vi "Catalytic Methanation #1.vi"() -> ()   [LabVIEW 2017]
uses:
  Halt S&THx.vi
  <vilib>/addons/control/pid/pid.llb/PID Advanced (DBL).vi
  <vilib>/addons/control/pid/NI_PID_pid.lvlib
panel:
  out "Last Time Write":dbl
  in  "Replace File":bool
  in  "Recording Increment (sec)":dbl=0.3 min=0.1 max=100.0 step=0.1 format="%#_13g"
  in  "Enable 5":bool
  in  "stop":bool
  out "error constant":errorcluster
  out "Inlet Valve":bool=TRUE
  out "Heater On?":bool
  in  "Td (Pressure)":dbl
  in  "Ti (Pressure)":dbl=0.01
  in  "Kc (Pressure)":dbl=-5.0
  in  "Td (Heater)":dbl caption="(min)"
  in  "Ti (Heater)":dbl=5.0 caption="(min)"
  in  "Kc (Heater)":dbl=1.0
  in  "Select GC Analysis Stream":enum32{"Reactor Feed", "Reactor Exhaust"}(radio)=enum."Reactor Exhaust"
  out "He Flowrate (SCCM)":dbl format="%.1f"
  out "H2 Flowrate (SCCM)":dbl format="%.2f"
  out "CO2 Flowrate (SCCM)":dbl format="%.2f"
  in  "He Setpoint (SCCM)":dbl min=0.0 max=200.0 format="%.1f"
  in  "H2 Setpoint (SCCM)":dbl min=0.0 max=50.0 format="%.2f"
  in  "Heater Switch":bool
  in  "CO2 Setpoint (SCCM)":dbl min=0.0 max=10.0 format="%.2f"
  in  "Temperature Setpoint (C)":dbl=20.0 min=0.0 max=325.0 format="%.1f"
  out "Reactor Temperature (C)":dbl format="%.2f"
  out "Heater Output (%)":dbl(slide) scale=0.0..100.0
  in  "Manual  Override (Temperature)":bool=TRUE
  in  "Set Manual  Heater Output (Temperature)":dbl(slide) scale=0.0..100.0
  in  "Reactor Pressure  Setpoint (psia)":dbl=18.4 min=0.0 max=30.0 format="%.1f"
  out "Reactor Pressure (psia)":dbl format="%.1f"
  out "Pressure Control Valve (%)":dbl(slide) scale=0.0..100.0
  in  "Manual Override (Pressure)":bool=TRUE
  in  "Set Manual Valve Position (Pressure)":dbl(slide)=50.0 scale=0.0..100.0
  # "Heater Power"
  # "Total Flow > 190 SCCM\nH2/CO2 > 3.85\nGC Sample Path: Reactor Exhaust"
  # "Heater Control"
  # "Gas Flow Rates (SCCM)"
  # "Setpoint"
  # "Actual"
  # "Hydrogen"
  # "Carbon Dioxide"
  # "Helium"
  # "Data Collection"
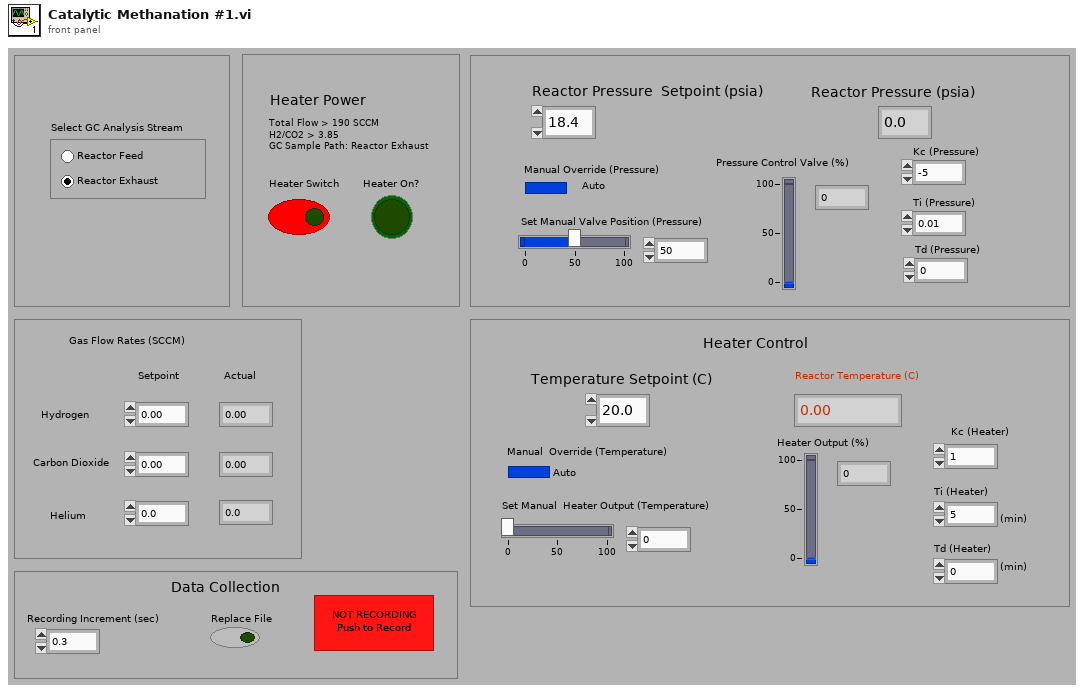
[diagram p1: front panel]
types:
  T1 = enum16{"open", "replace", "create", "open or create", "replace or create", "replace or create with confirmation"}
  T2 = cluster{"Kc (Heater)":dbl, "Ti (Heater)":dbl, "Td (Heater)":dbl}
  T3 = cluster{"Kc (Pressure)":dbl, "Ti (Pressure)":dbl, "Td (Pressure)":dbl}
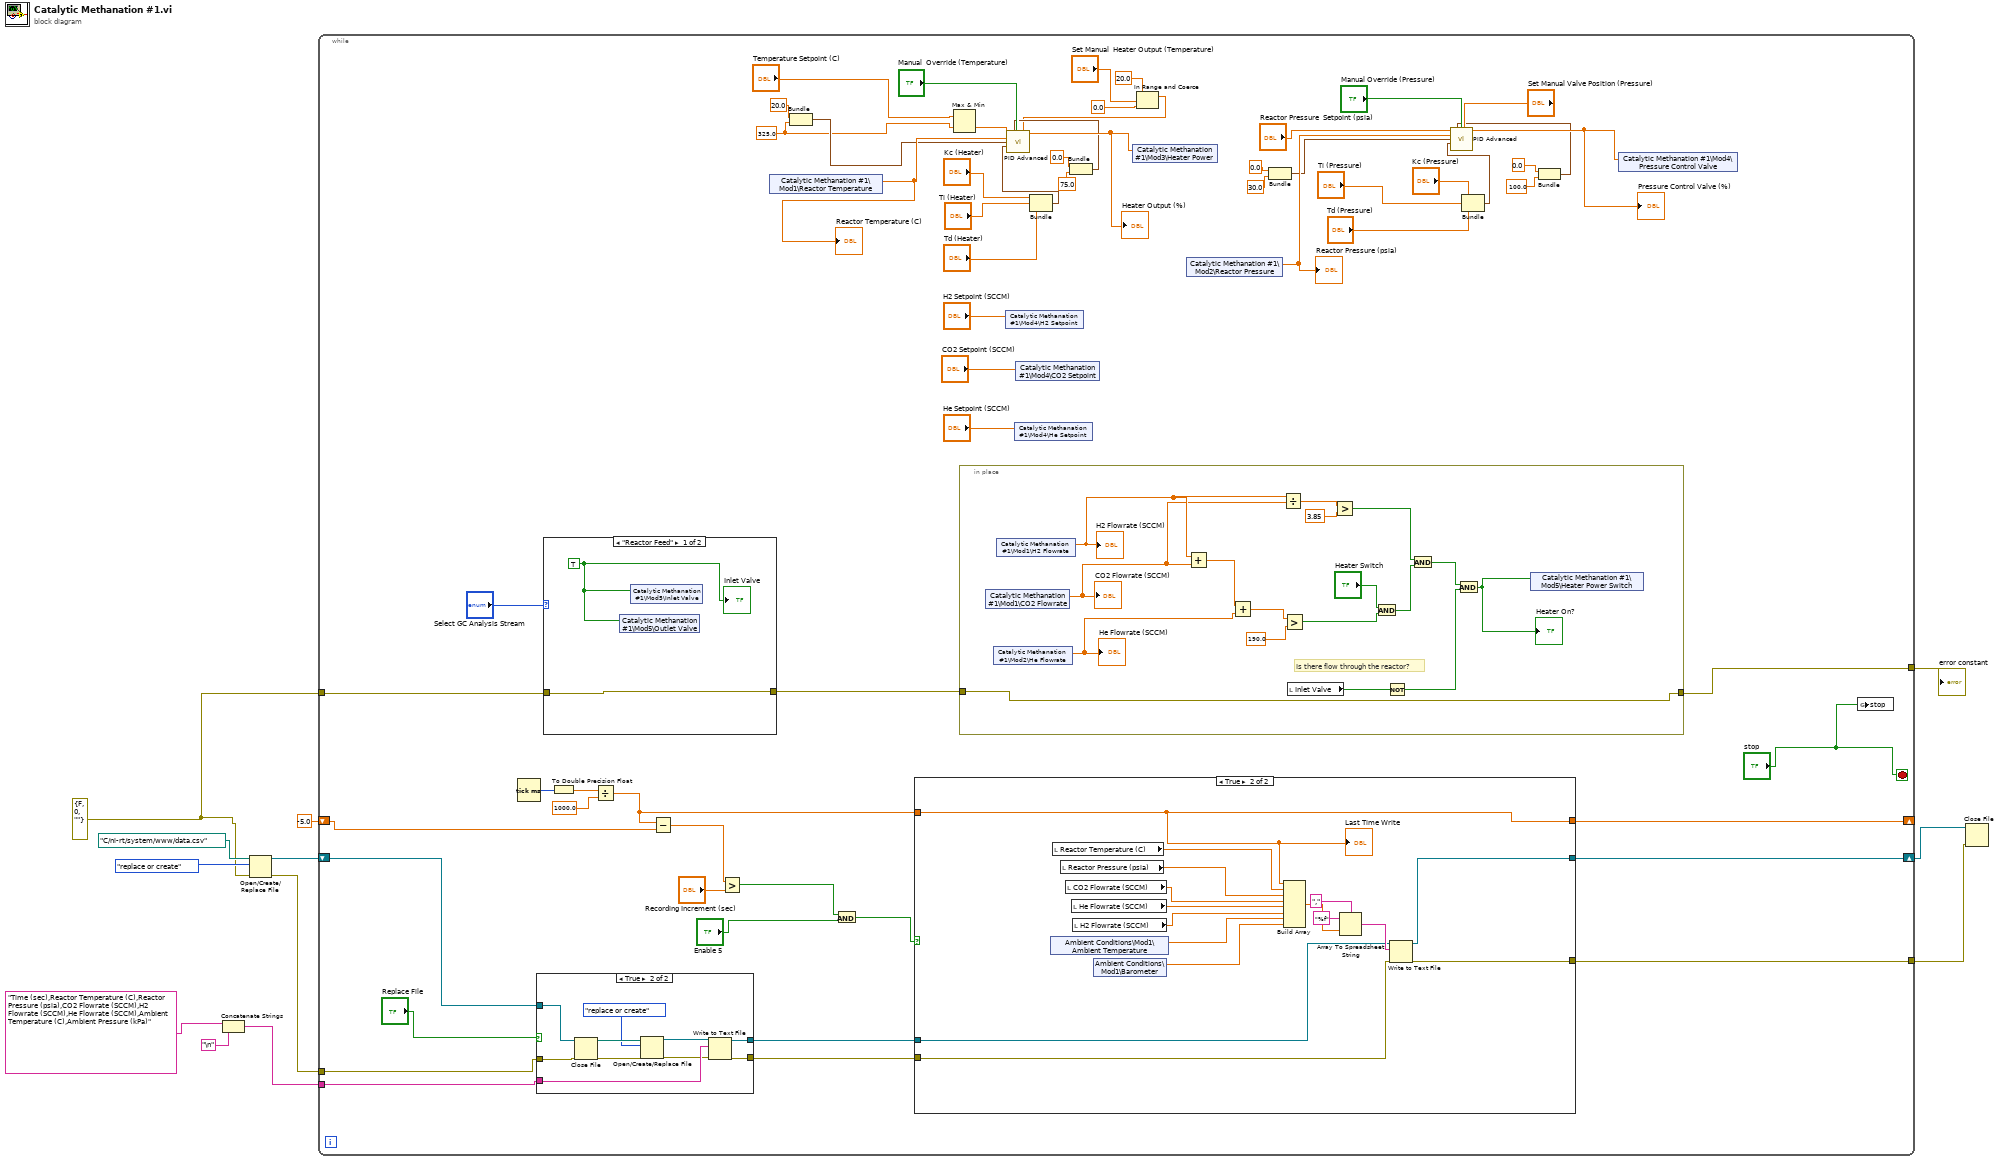
[diagram p0: block diagram]
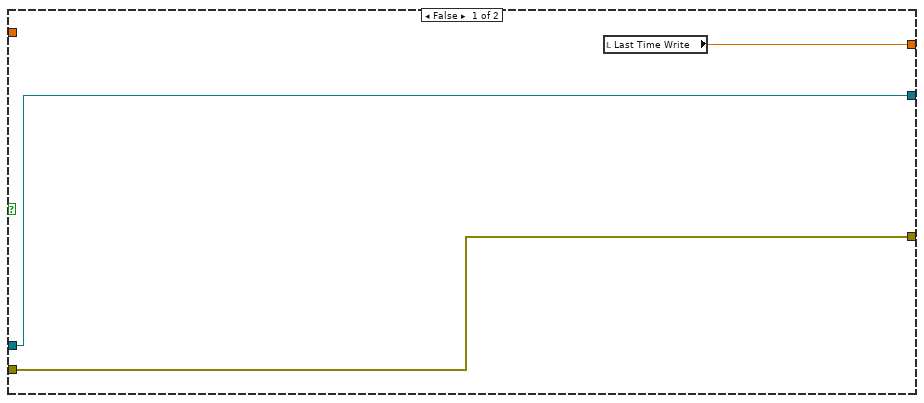
[diagram p2: hidden frame]
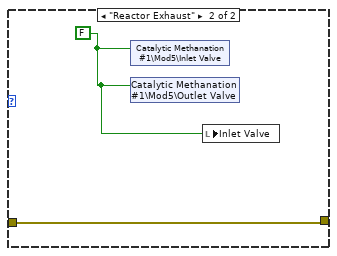
[diagram p4: hidden frame]
diagram:
  w9 = errorcluster {"status"=FALSE, "code"=0, "source"=""} ("error constant")
  n1 = Concatenate Strings("Time (sec),Reactor Temperature (C),Reactor Pressure (psia),CO2 Flowrate (SCCM),H2 Flowrate (SCCM),He Flowrate (SCCM),Ambient Temperature (C),Ambient Pressure (kPa)", "\n") -> (w4:string)
  n2 = Open/Create/Replace File(file path (use dialog)=path "C:/ni-rt/system/www/data.csv" ("Filename"), error in=w9, operation (0:open)=T1."replace or create") -> (refnum out=w8:refnum<file>, error out=w7:errorcluster)  [unwired: 3 in, 1 out]
  n3 = while {
    tunnel: w9 -> [w35]
    tunnel: [w33] -> w12
    shift-right: [w17] -> w1
    shift-left: w8 -> [w26]
    tunnel: w7 -> [w24]
    tunnel: w4 -> [w23]
    tunnel: [w18] -> w2
    shift-right: [w15] -> _
    shift-left: -5.0 ("Last Time Write") -> [w14]
    stop <- "stop" stop-if-true
    w49 = 325.0
    n4 = Tick Count (ms)() -> (millisecond timer value=w29:u32)
    n5 = case shown="True" "Replace File" {
      tunnel: w23 -> [_ w102]
      tunnel: w26 -> [w94 w100]
      tunnel: [w94 w99] -> w16
      tunnel: w24 -> [w93 w98]
      tunnel: [w93 w95] -> w19
      frame False {
      }
      frame True {
        n6 = Close File(refnum=w100, error in=w98) -> (path=w103:path, error out=w97:errorcluster)
        n7 = Open/Create/Replace File(file path (use dialog)=w103, error in=w97, operation (0:open)=T1."replace or create") -> (refnum out=w104:refnum<file>, error out=w96:errorcluster)  [unwired: 3 in, 1 out]
        n8 = Write to Text File(file (use dialog)=w104, text=w102, error in=w96) -> (refnum out=w99:refnum<file>, error out=w95:errorcluster)  [unwired: 1 in, 1 out]
      }
    }
    n9 = case shown="\"Reactor Feed\"" "Select GC Analysis Stream" {
      tunnel: [w122 w124] -> w34
      tunnel: w35 -> [w122 w124]
      frame "Reactor Feed" {
        w123 = TRUE ("Inlet Valve")
        n10 = shared-variable "Catalytic Methanation #1\\Mod5\\Outlet Valve"(w123) -> ()  [unwired: 1 in, 1 out]
        n11 = shared-variable "Catalytic Methanation #1\\Mod5\\Inlet Valve"(w123) -> ()  [unwired: 1 in, 1 out]
        "Inlet Valve" <- w123
      }
      frame "Reactor Exhaust" {
        w125 = FALSE
        n12 = shared-variable "Catalytic Methanation #1\\Mod5\\Inlet Valve"(w125) -> ()  [unwired: 1 in, 1 out]
        n13 = shared-variable "Catalytic Methanation #1\\Mod5\\Outlet Valve"(w125) -> ()  [unwired: 1 in, 1 out]
        n14 = local write "Inlet Valve"(w125) -> ()
      }
    }
    n15 = To Double Precision Float(number=w29) -> (double precision float=w28:dbl)
    n16 = Divide(x=w28, y=1000.0) -> (x/y=w20:dbl)
    n17 = Subtract(x=w20, y=w14) -> (x-y=w30:dbl)
    n18 = Greater?(x=w30, y="Recording Increment (sec)") -> (0:w21:bool)
    n19 = shared-variable "Catalytic Methanation #1\\Mod1\\Reactor Temperature"() -> (w59:dbl)  [unwired: 1 in, 1 out]
    "Reactor Temperature (C)" <- w59
    n20 = Bundle(20.0, w49) -> (w51:cluster{dbl, dbl})  [unwired: 1 in]
    n21 = And(x=w21, y="Enable 5") -> (x .and. y?=w13:bool)
    n22 = case shown="True" w13 {
      tunnel: w20 -> [_ w77]
      tunnel: w19 -> [w74 w82]
      tunnel: [w74 w81] -> w18
      tunnel: [w75 w80] -> w17
      tunnel: w16 -> [w75 w78]
      tunnel: [w76 w77] -> w15
      frame False {
        n23 = local read "Last Time Write"() -> (w76:dbl)
      }
      frame True {
        n24 = shared-variable "Ambient Conditions\\Mod1\\Ambient Temperature"() -> (w84:dbl)  [unwired: 1 in, 1 out]
        n25 = local read "Reactor Temperature (C)"() -> (w89:dbl)
        n26 = local read "Reactor Pressure (psia)"() -> (w88:dbl)
        n27 = local read "CO2 Flowrate (SCCM)"() -> (w87:dbl)
        n28 = local read "He Flowrate (SCCM)"() -> (w86:dbl)
        n29 = local read "H2 Flowrate (SCCM)"() -> (w85:dbl)
        n30 = shared-variable "Ambient Conditions\\Mod1\\Barometer"() -> (w83:dbl)  [unwired: 1 in, 1 out]
        n31 = Build Array(w77, w89, w88, w87, w86, w85, w84, w83) -> (w92:dbl[])
        n32 = Array To Spreadsheet String(delimiter (Tab)=",", array=w92, 3:"%f") -> (spreadsheet string=w79:string)
        n33 = Write to Text File(file (use dialog)=w78, text=w79, error in=w82) -> (refnum out=w80:refnum<file>, error out=w81:errorcluster)  [unwired: 1 in, 1 out]
        "Last Time Write" <- w77
      }
    }
    n34 = Max & Min(x="Temperature Setpoint (C)", y=w49) -> (min(x,y)=w41:dbl)  [unwired: 1 out]
    n35 = in-place {
      in-place-border: w34 -> [w105]
      in-place-border: [w105] -> w33
      # "Is there flow through the reactor?"
      n36 = shared-variable "Catalytic Methanation #1\\Mod1\\CO2 Flowrate"() -> (w114:dbl)  [unwired: 1 in, 1 out]
      "CO2 Flowrate (SCCM)" <- w114
      n37 = shared-variable "Catalytic Methanation #1\\Mod2\\He Flowrate"() -> (w121:dbl)  [unwired: 1 in, 1 out]
      "He Flowrate (SCCM)" <- w121
      n38 = shared-variable "Catalytic Methanation #1\\Mod1\\H2 Flowrate"() -> (w115:dbl)  [unwired: 1 in, 1 out]
      "H2 Flowrate (SCCM)" <- w115
      n39 = Add(x=w115, y=w114) -> (x+y=w120:dbl)
      n40 = Add(x=w120, y=w121) -> (x+y=w119:dbl)
      n41 = Divide(x=w115, y=w114) -> (x/y=w113:dbl)
      n42 = Greater?(x=w119, y=190.0) -> (0:w117:bool)
      n43 = local read "Inlet Valve"() -> (w107:bool)
      n44 = Greater?(x=w113, y=3.85) -> (0:w110:bool)
      n45 = And(x="Heater Switch", y=w117) -> (x .and. y?=w111:bool)
      n46 = Not(x=w107) -> (.not. x?=w106:bool)
      n47 = And(x=w110, y=w111) -> (x .and. y?=w109:bool)
      n48 = And(x=w109, y=w106) -> (x .and. y?=w108:bool)
      "Heater On?" <- w108
      n49 = shared-variable "Catalytic Methanation #1\\Mod5\\Heater Power Switch"(w108) -> ()  [unwired: 1 in, 1 out]
    }
    n50 = shared-variable "Catalytic Methanation #1\\Mod4\\H2 Setpoint"("H2 Setpoint (SCCM)") -> ()  [unwired: 1 in, 1 out]
    n51 = shared-variable "Catalytic Methanation #1\\Mod4\\He Setpoint"("He Setpoint (SCCM)") -> ()  [unwired: 1 in, 1 out]
    n52 = shared-variable "Catalytic Methanation #1\\Mod4\\CO2 Setpoint"("CO2 Setpoint (SCCM)") -> ()  [unwired: 1 in, 1 out]
    n53 = Bundle("Kc (Heater)"="Kc (Heater)", "Ti (Heater)"="Ti (Heater)", "Td (Heater)"="Td (Heater)") -> (w68:T2)  [unwired: 1 in]
    n54 = Bundle(0.0, 75.0) -> (w53:cluster{dbl, dbl})  [unwired: 1 in]
    n55 = In Range and Coerce(upper limit=20.0, x="Set Manual  Heater Output (Temperature)", lower limit=0.0) -> (coerced(x)=w39:dbl)  [unwired: 1 out]
    n56 = call-poly <vilib>:"PID Advanced.vi"("setpoint"=w41, "output range"=w53, "auto? (T)"="Manual  Override (Temperature)", "manual control"=w39, "process variable"=w59, "setpoint range"=w51, "PID gains"=w68) -> ("output"=w61:dbl)  [unwired: 7 in, 1 out]
    "Heater Output (%)" <- w61
    n57 = shared-variable "Catalytic Methanation #1\\Mod3\\Heater Power"(w61) -> ()  [unwired: 1 in, 1 out]
    n58 = shared-variable "Catalytic Methanation #1\\Mod2\\Reactor Pressure"() -> (w70:dbl)  [unwired: 1 in, 1 out]
    "Reactor Pressure (psia)" <- w70
    n59 = Bundle(0.0, 30.0) -> (w47:cluster{dbl, dbl})  [unwired: 1 in]
    n60 = Bundle("Kc (Pressure)"="Kc (Pressure)", "Ti (Pressure)"="Ti (Pressure)", "Td (Pressure)"="Td (Pressure)") -> (w69:T3)  [unwired: 1 in]
    n61 = Bundle(0.0, 100.0) -> (w44:cluster{dbl, dbl})  [unwired: 1 in]
    n62 = call-poly <vilib>:"PID Advanced.vi"("setpoint"="Reactor Pressure  Setpoint (psia)", "output range"=w44, "auto? (T)"="Manual Override (Pressure)", "manual control"="Set Manual Valve Position (Pressure)", "process variable"=w70, "setpoint range"=w47, "PID gains"=w69) -> ("output"=w73:dbl)  [unwired: 7 in, 1 out]
    "Pressure Control Valve (%)" <- w73
    n63 = shared-variable "Catalytic Methanation #1\\Mod4\\Pressure Control Valve"(w73) -> ()  [unwired: 1 in, 1 out]
    n64 = global write "Halt S&THx.vi" "stop"("stop") -> ()
  }
  "error constant" <- w12
  n65 = Close File(refnum=w1, error in=w2) -> ()  [unwired: 2 out]
